vi "read_params.vi"(8 "error in (no error)":errorcluster, 11 "LinearSVR in":refnum<class "LinearSVR.lvclass">) -> (0 "error out":errorcluster, 2 "params":T1={"epsilon"=0.0, "tol"=0.0001, "C"=1.0, "loss"="epsilon_insensitive", "fit_intercept"=TRUE, "intercept_scaling"=1.0, "dual"=TRUE, "verbose"=0.0, "random_state"=0.0, "max_iter"=1000.0}, 3 "LinearSVR out":refnum<class "LinearSVR.lvclass">)   [LabVIEW 2020, in "LinearSVR.lvclass"]
uses:
  LinearSVR.lvclass
  Controls/linear_svr_params.ctl
  LinearSVR.lvclass/LinearSVR.ctl
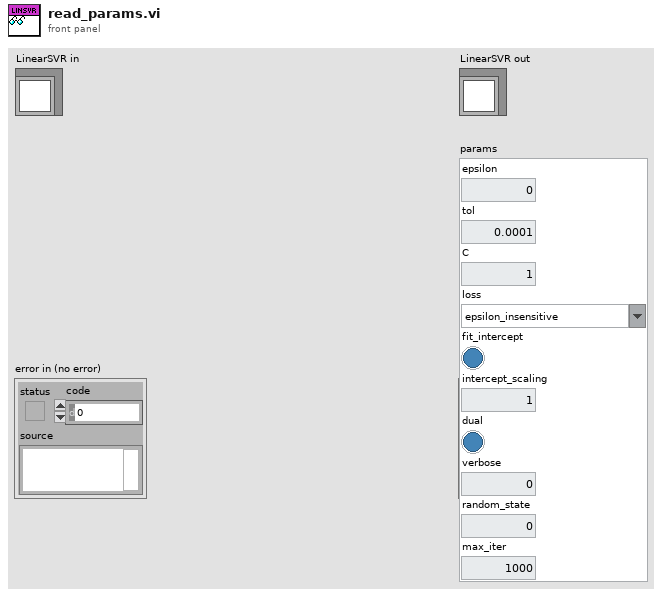
[diagram p1: front panel]
types:
  T1 = typedef "linear_svr_params.ctl" = cluster{"epsilon":dbl, "tol":dbl, "C":dbl, "loss":string, "fit_intercept":bool, "intercept_scaling":dbl, "dual":bool, "verbose":dbl, "random_state":dbl, "max_iter":dbl}
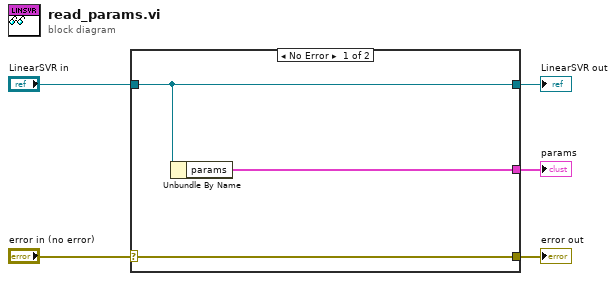
[diagram p0: block diagram]
diagram:
  n1 = case shown="No Error" "error in (no error)" {
    selector: "error in (no error)" -> [w8 w9]
    tunnel: [w8 w9] -> w4
    tunnel: [w7 w10] -> w2
    tunnel: "LinearSVR in" -> [w7 w10]
    tunnel: [w6 _] -> w1
    frame No Error {
      n2 = Unbundle By Name(w7) -> ("params"=w6:T1)
    }
    frame Error {
    }
  }
  "error out" <- w4
  "LinearSVR out" <- w2
  "params" <- w1
